vi "Send ShowPanel.vi"(7 "Message Priority (Normal)":T1=enum."Normal", 8 "error in (no error)":errorcluster, 11 "Message Enqueuer":refnum<class "Message Enqueuer.lvclass">) -> (0 "error out":errorcluster, 2 "FP.NativeWindow":u64, 3 "Message Enqueuer out":refnum<class "Message Enqueuer.lvclass">)   [LabVIEW 2025, in "Task_Abstr.lvlib" / "ShowPanel Msg.lvclass"]
doc: "This VI sends the message to an actor."
uses:
  ShowPanel Msg.lvclass
  <vilib>/ActorFramework/Message Enqueuer/Message Enqueuer.lvclass
  <vilib>/ActorFramework/Message Enqueuer/Message Priority.ctl
  <vilib>/ActorFramework/Message Enqueuer/Message Enqueuer.lvclass/Message Enqueuer.ctl
  <vilib>/ActorFramework/Message Priority Queue/Priority Enqueue.vi
  ShowPanel Msg.lvclass/ShowPanel Msg.ctl
  C:/Program Files (x86)/National Instruments/LabVIEW 2025/vi.lib/ActorFramework/Message/Message.lvclass
  D:/Hardware/DAQ/DAQ_Abstr/Task_Abstr/Task_Abstr Messages/ShowPanel Msg/ShowPanel Msg.lvclass
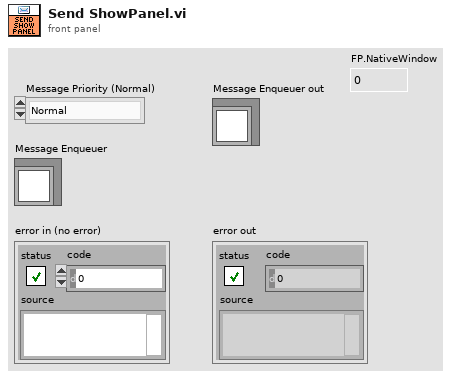
[diagram p1: front panel]
types:
  T1 = typedef "Actor Framework.lvlib/Message Enqueuer.lvclass/Message Priority.ctl" = enum16{"Low", "Normal", "High"}
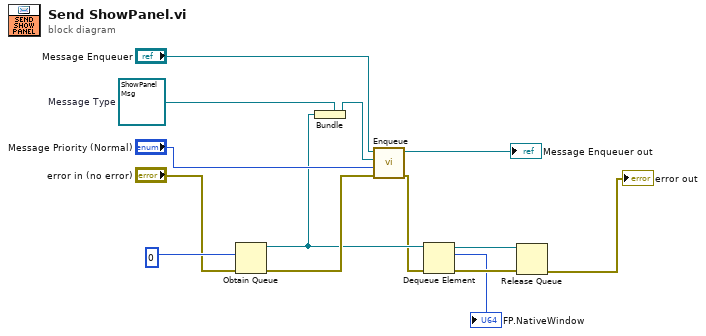
[diagram p0: block diagram]
diagram:
  w13 = refnum<class "ShowPanel Msg.lvclass"> refnum  # Message Type
  n1 = Obtain Queue(element data type=u64 0 ("FP.NativeWindow"), error in (no error)="error in (no error)") -> (queue out=w6:refnum<queue>, error out=w7:errorcluster)  [unwired: 3 in, 1 out]
  n2 = Bundle(cluster=w13, w6) -> (w9:refnum<class "ShowPanel Msg.lvclass">)
  n3 = call <vilib>:"Enqueue.vi"("error in (no error)"=w7, "Message Priority (Normal)"="Message Priority (Normal)", "Message"=w9, "Message Enqueuer in"="Message Enqueuer") -> ("error out"=w5:errorcluster, "Message Enqueuer out"=→"Message Enqueuer out":refnum<class "Message Enqueuer.lvclass">)  [unwired: 6 in]
  n4 = Dequeue Element(queue=w6, error in (no error)=w5) -> (queue out=w4:refnum<queue>, element=→"FP.NativeWindow":u64, error out=w3:errorcluster)  [unwired: 1 in, 1 out]
  n5 = Release Queue(queue=w4, error in (no error)=w3) -> (error out=→"error out":errorcluster)  [unwired: 1 in, 2 out]
